vi "ex2_basic_modified.vi"() -> ()   [LabVIEW 2012]
panel:
  out "error out 2":errorcluster
  in  "Take Image":bool
  out "Image":T1(plugin-control)
  out "error out":errorcluster
  in  "error in (no error)":errorcluster
  in  "stop":bool
  out "Preview Window":picture
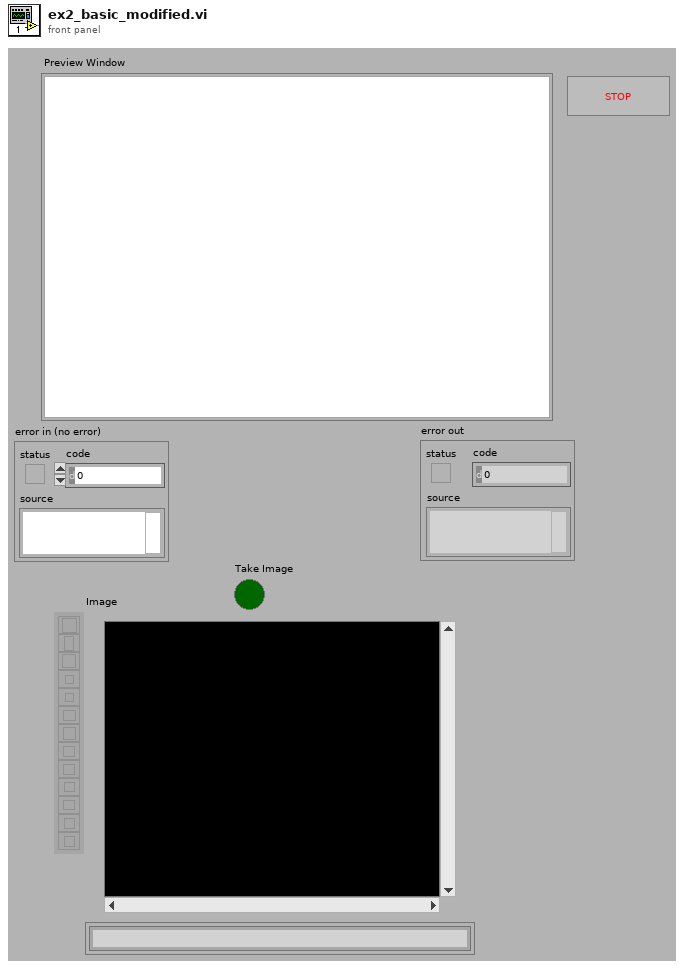
[diagram p1: front panel]
types:
  T1 = typedef "IMAQ Image.ctl" = refnum<image>
  T2 = typedef "Image Type" = u32
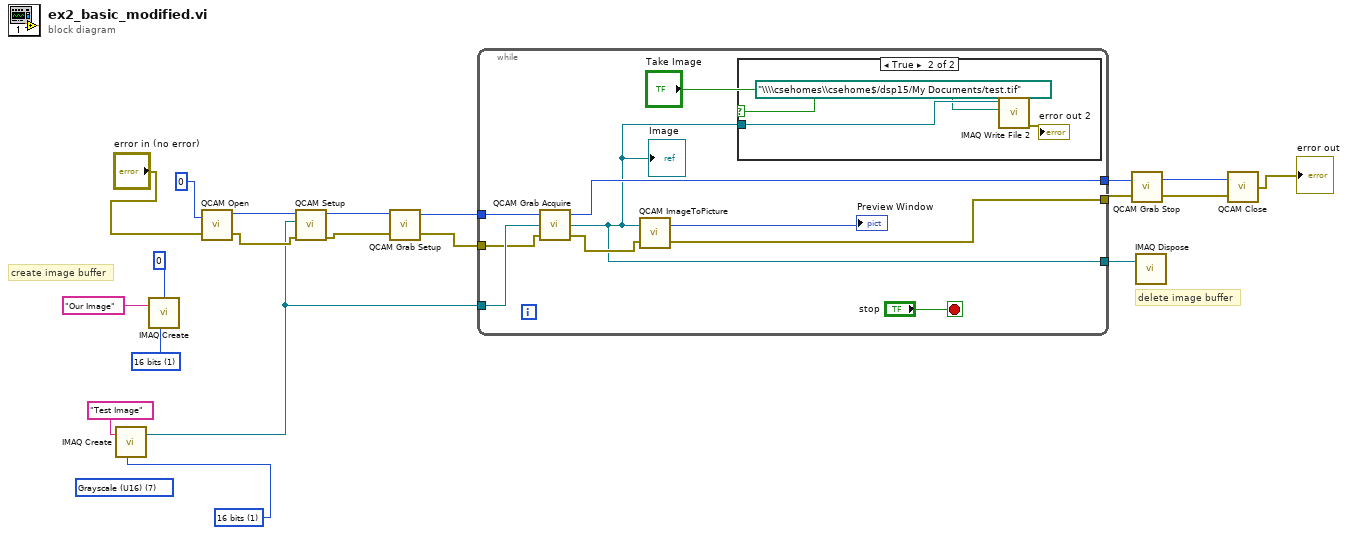
[diagram p0: block diagram]
diagram:
  w2 = u32 1 items=["8 bits", "16 bits"] ("Image Type")
  (unwired) T2 7 items=["Grayscale (U8)", "Grayscale (I16)", "Grayscale (SGL)", "Complex (CSG)", "RGB (U32)", "HSL (U32)", "RGB (U64)", "Grayscale (U16)"] ("Image Type")
  w20 = u32 1 items=["8 bits", "16 bits"] ("Image Type")
  # "create image buffer"
  # "delete image buffer"
  n1 = call "IMAQ Create"("Image Name"="Test Image", "Image Type"=w2) -> ("New Image"=w1:T1)  [unwired: 3 in, 1 out]
  n2 = call "IMAQ Create"("Border Size"=0, "Image Name"="Our Image", "Image Type"=w20) -> ()  [unwired: 1 in, 3 out]
  n3 = call "QCAM Open.vi"("error in (no error)"="error in (no error)", "cameraId"=0) -> ("error out"=w11:errorcluster, "cameraId out"=w15:u32)
  n4 = call "QCAM Setup.vi"("error in (no error)"=w11, "Image"=w1, "cameraId"=w15) -> ("error out"=w10:errorcluster, "cameraId out"=w16:u32)  [unwired: 3 in, 4 out]
  n5 = call "QCAM Grab Setup.vi"("error in (no error)"=w10, "cameraId"=w16) -> ("error out"=w9:errorcluster, "cameraId out"=w19:u32)
  n6 = while {
    tunnel: [w21] -> w13
    tunnel: w1 -> [w26]
    tunnel: w19 -> [w28]
    tunnel: [w29] -> w18
    tunnel: w9 -> [w25]
    tunnel: [w23] -> w6
    stop <- "stop" stop-if-true
    n7 = call "QCAM Grab Acquire.vi"("error in (no error)"=w25, "Image"=w26, "cameraId"=w28) -> ("error out"=w24:errorcluster, "Image Out"=w21:T1, "cameraId out"=w29:u32)
    "Image" <- w21
    n8 = call <userlib>:"QCAM ImageToPicture.vi"("error in (no error)"=w24, "Image"=w21) -> ("error out"=w23:errorcluster, "Picture Out"=→"Preview Window":picture)
    n9 = case shown="True" "Take Image" {
      tunnel: w21 -> [_ w33]
      frame False {
      }
      frame True {
        n10 = call-poly "IMAQ Write File 2"("File Path"=path "\\\\csehomes\\csehome$/dsp15/My Documents/test.tif", "Image"=w33) -> ("error out"=→"error out 2":errorcluster)  [unwired: 8 in, 1 out]
      }
    }
  }
  n11 = call "QCAM Grab Stop.vi"("error in (no error)"=w6, "cameraId"=w18) -> ("error out"=w5:errorcluster, "cameraId Out"=w14:u32)
  n12 = call "IMAQ Dispose"("Image"=w13) -> ()  [unwired: 2 in, 4 out]
  n13 = call "QCAM Close.vi"("error in (no error)"=w5, "cameraId"=w14) -> ("error out"=→"error out":errorcluster)
